vi "Day 3 (Part Two).vi"() -> ()   [LabVIEW 2021]
panel:
  out "sum":i32
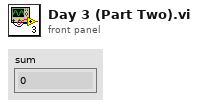
[diagram p1: front panel]
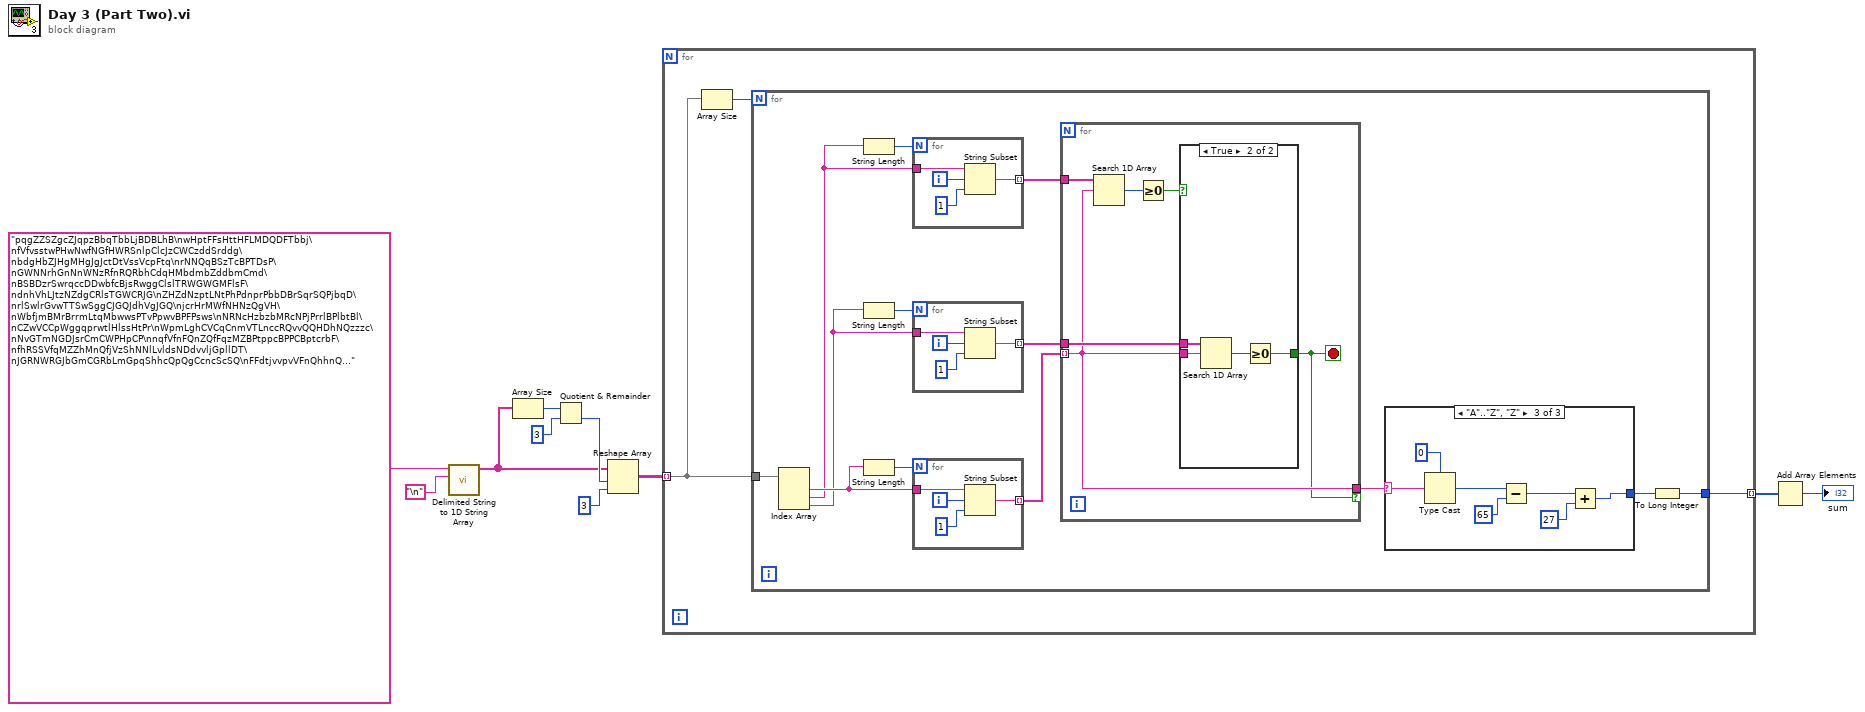
[diagram p0: block diagram]
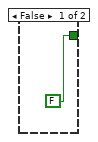
[diagram p2: hidden frame]
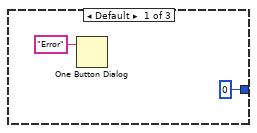
[diagram p3: hidden frame]
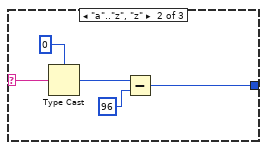
[diagram p4: hidden frame]
diagram:
  n1 = call <vilib>:"Delimited String to 1D String Array.vi"("delimiter"="\n", "delimited string"="pqgZZSZgcZJqpzBbqTbbLjBDBLhB\nwHptFFsHttHFLMDQDFTbbj\nfVfvsstwPHwNwfNGfHWRSnlpClcJzCWCzddSrddg\nbdgHbZJHgMHgJgJctDtVssVcpFtq\nrNNQqBSzTcBPTDsP\nGWNNrhGnNnWNzRfnRQRbhCdqHMbdmbZddbmCmd\nBSBDzrSwrqccDDwbfcBjsRwggClslTRWGWGMFlsF\ndnhVhLJtzNZdgCRlsTGWCRJG\nZHZdNzptLNtPhPdnprPbbDBrSqrSQPjbqD\nrlSwlrGvwTTSwSggCJGQJdhVgJGQ\njcrHrMWfNHNzQgVH\nWbfjmBMrBrrmLtqMbwwsPTvPpwvBPFPsws\nNRNcHzbzbMRcNPjPrrlBPlbtBl\nCZwVCCpWggqprwtlHlssHtPr\nWpmLghCVCqCnmVTLnccRQvvQQHDhNQzzzc\nNvGTmNGDJsrCmCWPHpCP\nnqfVfnFQnZQfFqzMZBPtppcBPPCBptcrbF\nfhRSSVfqMZZhMnQfjVzShNNlLvldsNDdvvljGpllDT\nJGRNWRGJbGmCGRbLmGpqShhcQpQgCcncScSQ\nFFdtjvvpvVFnQhhnQ...") -> ("string array"=w1:string[])  [unwired: 9 in]
  n2 = Array Size(array=w1) -> (size(s)=w5:i32)
  n3 = Quotient & Remainder(x=w5, y=3) -> (floor(x/y)=w4:i32)  [unwired: 1 out]
  n4 = Reshape Array(w1, w4, 3 ("dimension size")) -> (w2:string[][])
  n5 = for {
    tunnel: [w12] -> w10 mode=indexing
    tunnel: w2 -> [w11] mode=indexing
    n6 = Array Size(array=w11) -> (size(s)=w13:i32)
    n7 = for {
      N: w13 -> [_]
      tunnel: w11 -> [w24]
      tunnel: [w25] -> w12
      n8 = Index Array(array=w24) -> (element #1=w22:string, element #2=w20:string, element #3=w18:string)  [unwired: 3 in]
      n9 = String Length(string=w20) -> (length=w19:i32)
      n10 = String Length(string=w18) -> (length=w17:i32)
      n11 = String Length(string=w22) -> (length=w23:i32)
      n12 = for {
        N: w19 -> [_]
        tunnel: w20 -> [w34]
        tunnel: [w31] -> w16 mode=indexing
        i -> [w32]
        n13 = String Subset(string=w34, offset (0)=w32, length (rest)=1 ("length (rest)")) -> (substring=w31:string)
      }
      n14 = for {
        N: w17 -> [_]
        tunnel: w18 -> [w30]
        tunnel: [w27] -> w15 mode=indexing
        i -> [w28]
        n15 = String Subset(string=w30, offset (0)=w28, length (rest)=1 ("length (rest)")) -> (substring=w27:string)
      }
      n16 = for {
        N: w23 -> [_]
        tunnel: [w36] -> w21 mode=indexing
        tunnel: w22 -> [w35]
        i -> [w37]
        n17 = String Subset(string=w35, offset (0)=w37, length (rest)=1 ("length (rest)")) -> (substring=w36:string)
      }
      n18 = for {
        tunnel: w21 -> [w40] mode=indexing
        tunnel: w16 -> [w44]
        tunnel: w15 -> [w42]
        tunnel: [w40] -> w14 if=w39
        stop <- w39 stop-if-true
        n19 = Search 1D Array(1D array=w44, element=w40) -> (index of element=w43:i32)  [unwired: 1 in]
        n20 = Greater Or Equal To 0?(x=w43) -> (x >= 0?=w41:bool)
        n21 = case shown="True" w41 {
          tunnel: w42 -> [_ w48]
          tunnel: w40 -> [_ w47]
          tunnel: [FALSE w46] -> w39
          frame False {
          }
          frame True {
            n22 = Search 1D Array(1D array=w48, element=w47) -> (index of element=w49:i32)  [unwired: 1 in]
            n23 = Greater Or Equal To 0?(x=w49) -> (x >= 0?=w46:bool)
          }
        }
      }
      n24 = case shown="\"A\"..\"Z\", \"Z\"" w14 {
        selector: w14 -> [_ w52 w60]
        tunnel: [u8 0 w54 w57] -> w26
        frame Default {
          n25 = One Button Dialog(message="Error") -> ()  [unwired: 1 in, 1 out]
        }
        frame "a".."z", "z" {
          n26 = Type Cast(type=u8 0, x=w52) -> (*(type *) &x=w53:u8)
          n27 = Subtract(x=w53, y=u8 96) -> (x-y=w54:u8)
        }
        frame "A".."Z", "Z" {
          n28 = Type Cast(type=u8 0, x=w60) -> (*(type *) &x=w61:u8)
          n29 = Subtract(x=w61, y=u8 65) -> (x-y=w59:u8)
          n30 = Add(x=w59, y=u8 27) -> (x+y=w57:u8)
        }
      }
      n31 = To Long Integer(number=w26) -> (32bit integer=w25:i32)
    }
  }
  n32 = Add Array Elements(numeric array=w10) -> (sum=→"sum":i32)
